vi "Norm Vector Calcul.vi"(10 "Gamma":dbl format="%#_13g", 11 "Velocity in":cluster{"x":dbl, "y":dbl}={"x"=10.0, "y"=10.0}) -> (2 "Vector u11/22":dbl, 3 "Vector u21/12":dbl)   [LabVIEW 2024, in "Game Board.lvclass"]
doc: "MIT Licence\nCopyright (c) 2024 David Grollier"
uses:
  Game Board.lvclass
  <vilib>/Analysis/_algsub.llb/Vector Norm Type.ctl
  <vilib>/Analysis/_algsub.llb/Real Vector Norm.vi
  <vilib>/Analysis/NI_AALPro.lvlib
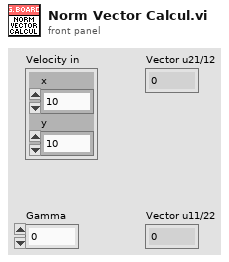
[diagram p1: front panel]
types:
  T1 = typedef "NI_AALPro.lvlib/Vector Norm Type.ctl" = u16
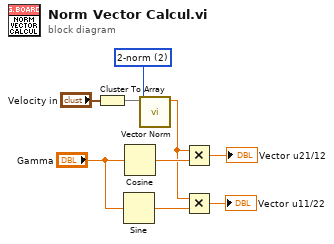
[diagram p0: block diagram]
diagram:
  w7 = T1 2 items=["1-norm"=1, "2-norm"=2, "Inf-norm"=3, "-Inf-norm"=4, "User Defined"=5] ("norm type")
  n1 = Cluster To Array(cluster="Velocity in") -> (array=w8:dbl[])
  n2 = Sine(x="Gamma") -> (sin(x)=w3:dbl)
  n3 = Cosine(x="Gamma") -> (cos(x)=w6:dbl)
  n4 = call-poly <vilib>:"Vector Norm.vi"("norm type"=w7, "Input Vector"=w8) -> ("norm"=w4:dbl)  [unwired: 8 in, 1 out]
  n5 = Multiply(x=w4, y=w6) -> (x*y=→"Vector u21/12":dbl)
  n6 = Multiply(x=w4, y=w3) -> (x*y=→"Vector u11/22":dbl)
